vi "Load Help File.vi"(8 "error in (no error)":errorcluster, 9 "HTML File to Load":string="MainPage_J1939.html", 11 "Browser":refnum<k7>(container)) -> (0 "error out":errorcluster)   [LabVIEW 2025, in "Runtime Configuration Support Example System Explorer.lvlib"]
doc: "Loads the specified HTML page from the CHM into the browser"
uses:
  Runtime Configuration Support Example System Explorer.lvlib
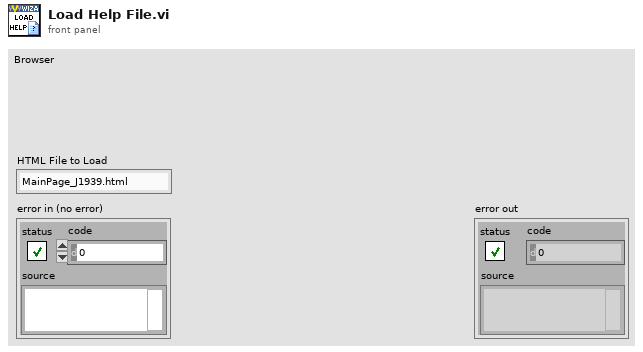
[diagram p1: front panel]
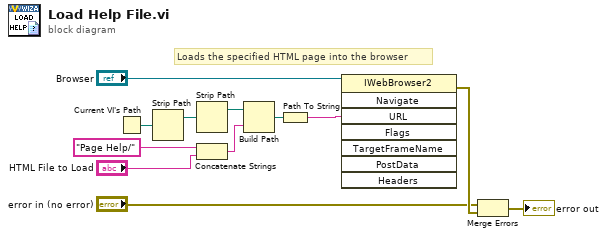
[diagram p0: block diagram]
diagram:
  # "Loads the specified HTML page into the browser"
  n1 = Current VI's Path() -> (path=w12:path)
  n2 = Strip Path(path=w12) -> (stripped path=w11:path)  [unwired: 1 out]
  n3 = Strip Path(path=w11) -> (stripped path=w9:path)  [unwired: 1 out]
  n4 = Concatenate Strings("Page Help/" ("string"), "HTML File to Load") -> (w2:string)
  n5 = Build Path(base path=w9, name or relative path=w2) -> (appended path=w10:path)
  n6 = Path To String(path=w10) -> (string=w1:string)
  n7 = invoke class="IWebBrowser2" method="Navigate"(reference="Browser", "URL"=w1) -> (error out=w7:errorcluster)  [unwired: 6 in, 7 out]
  n8 = Merge Errors("error in (no error)", w7) -> (→"error out":errorcluster)
